vi "Run Bfr Tx - Handle Transmit.vi"(6 "Bytes to Transmit":i32, 7 "Echo Resources in":T1, 8 "error in (no error)":errorcluster, 9 "Runtime Resources":T5={"Connection ID"=refnum, "Transmit Option"=enum."Always", "Destination IP Address"=0, "Destination Port"=0, "Multicast IP Address"=0, "TTL"=0, "Multicast"=FALSE, "Port as Channel"=FALSE, "ExecutionConfig"={"Loop Period"=0, "RT Loop Period"=-2, "Untimed Period"=0, "Target Processor"=0, "Priority"=0, "Thread Management"=enum."Untimed (Default)"}}, 10 "Buffer Resources":T3 {"Data Buffer" format="%016x"}, 11 "Buffer Option Support in":T9) -> (0 "error out":errorcluster, 4 "Tx Packet":string, 5 "Echo Resources out":T1)   [LabVIEW 2019, in "UDP-Custom-Device Engine.lvlib"]
uses:
  UDP-Custom-Device Engine.lvlib
  Types/Engine - Buffered Tx Buffer Option Support.ctl
  Shared/Types/Shared - Transmit Buffer Options.ctl
  Shared/Types/Shared - Transmit Sim Options.ctl
  Types/Engine - Tx Runtime Resources.ctl
  Shared/Types/Shared - Transmit Flag Options.ctl
  Types/Engine - Execution Config.ctl
  Shared/Types/Shared - Thread Management.ctl
  Types/Engine - Buffer Resources.ctl
  Shared/Types/Shared - Pointer Encoding.ctl
  Types/Engine - Tx Echo Resources.ctl
  Shared/Types/Shared - Transmit Echo Options.ctl
  <vilib>/NI VeriStand/VeriStand Data/Pointer Operations/Pointer.In-Place Read (1D U8).vi
  <vilib>/NI VeriStand/VeriStand Data/Pointer Operations/Pointer.Read.vi
  <vilib>/NI VeriStand/VeriStand Data/Pointer Operations/Pointer.Read (I32).vi
  <vilib>/NI VeriStand/VeriStand Data/Pointer Operations/Pointer.Read (U16).vi
  <vilib>/NI VeriStand/VeriStand Data/Pointer Operations/Pointer.In-Place Read (I32).vi
  <vilib>/NI VeriStand/VeriStand Data/Pointer Operations/Pointer.In-Place Read (U16).vi
  <vilib>/NI VeriStand/VeriStand Data/VeriStand Data.lvlib
  Shared/UDP-Custom-Device Shared.lvlib
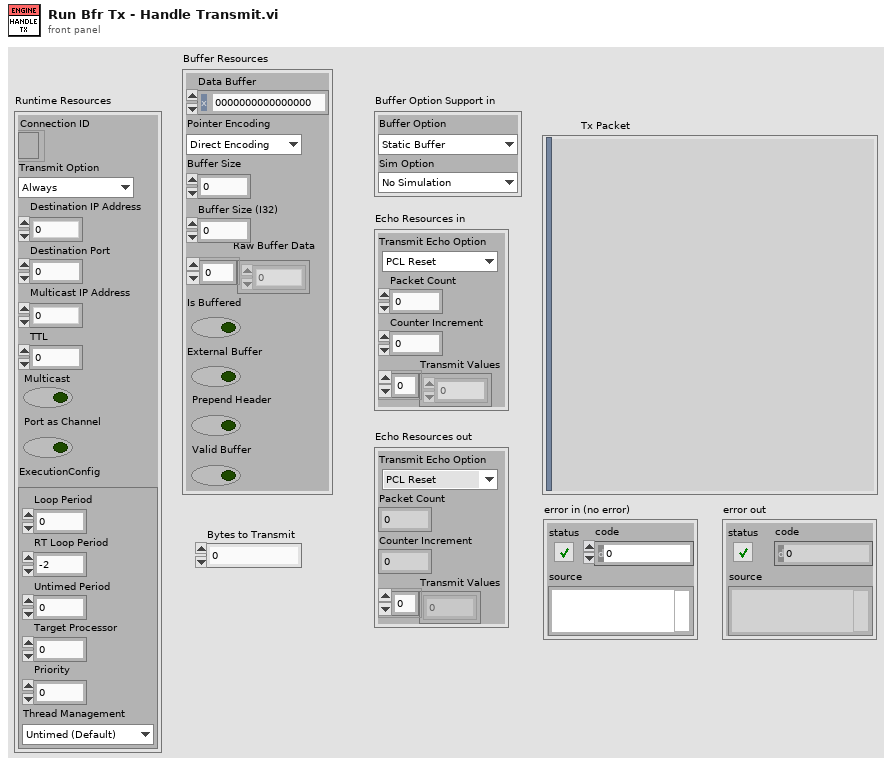
[diagram p1: front panel]
types:
  T1 = typedef "UDP-Custom-Device Engine.lvlib/Engine - Tx Echo Resources.ctl" = cluster{"Transmit Echo Option":T2, "Packet Count":dbl, "Counter Increment":dbl, "Transmit Values":dbl[]}
  T2 = typedef "UDP-Custom-Device Shared.lvlib/Shared - Transmit Echo Options.ctl" = enum16{"PCL Reset", "Counter", "Mirror"}
  T3 = typedef "UDP-Custom-Device Engine.lvlib/Engine - Buffer Resources.ctl" = cluster{"Data Buffer":u64, "Pointer Encoding":T4, "Buffer Size":u64, "Buffer Size (I32)":i32, "Raw Buffer Data":u8[], "Is Buffered":bool, "External Buffer":bool, "Prepend Header":bool, "Valid Buffer":bool}
  T4 = typedef "UDP-Custom-Device Shared.lvlib/Shared - Pointer Encoding.ctl" = enum16{"Direct Encoding", "Conversion Encoding"}
  T5 = typedef "UDP-Custom-Device Engine.lvlib/Engine - Tx Runtime Resources.ctl" = cluster{"Connection ID":refnum<k16>, "Transmit Option":T6, "Destination IP Address":u32, "Destination Port":u16, "Multicast IP Address":u32, "TTL":u16, "Multicast":bool, "Port as Channel":bool, "ExecutionConfig":T7}
  T6 = typedef "UDP-Custom-Device Shared.lvlib/Shared - Transmit Flag Options.ctl" = enum16{"Always", "One-Shot", "Toggle"}
  T7 = typedef "UDP-Custom-Device Engine.lvlib/Engine - Execution Config.ctl" = cluster{"Loop Period":i64, "RT Loop Period":i64, "Untimed Period":u32, "Target Processor":i32, "Priority":i32, "Thread Management":T8}
  T8 = typedef "UDP-Custom-Device Shared.lvlib/Shared - Thread Management.ctl" = enum16{"Untimed (Default)", "Timed (High Priority)"}
  T9 = typedef "UDP-Custom-Device Engine.lvlib/Engine - Buffered Tx Buffer Option Support.ctl" = cluster{"Buffer Option":T10, "Sim Option":T11}
  T10 = typedef "UDP-Custom-Device Shared.lvlib/Shared - Transmit Buffer Options.ctl" = enum16{"Static Buffer", "FIFO Buffer", "FIFO Buffer + Port"}
  T11 = typedef "UDP-Custom-Device Shared.lvlib/Shared - Transmit Sim Options.ctl" = enum16{"No Simulation", "Counter", "Full Buffer", "FIFO Test", "FIFO + Port Test"}
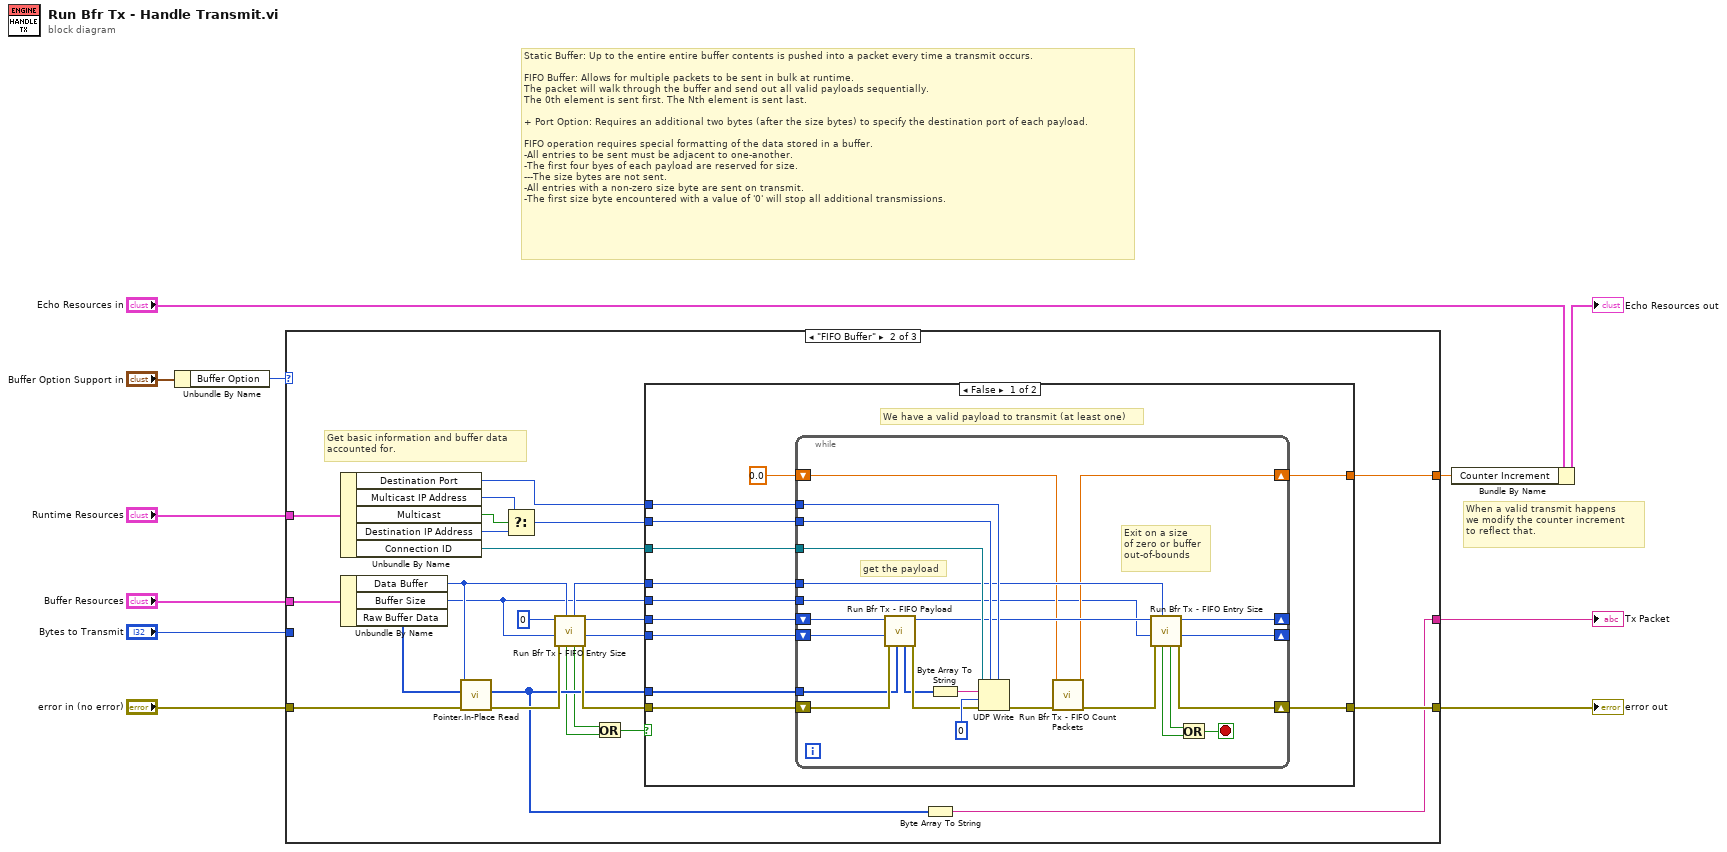
[diagram p0: block diagram]
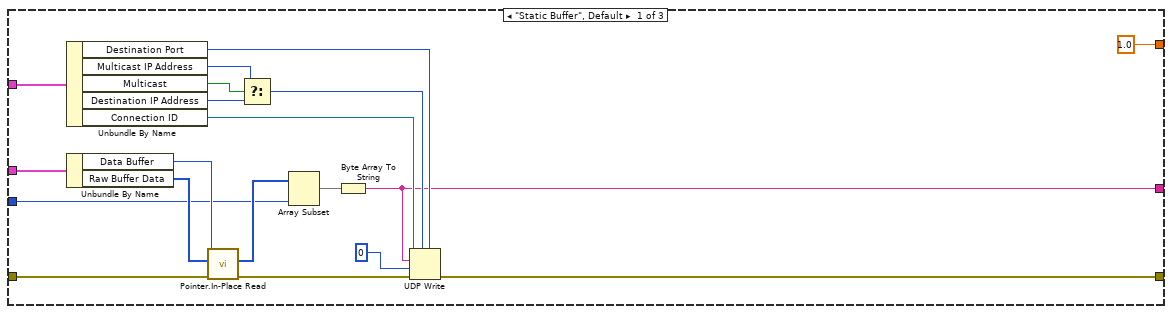
[diagram p2: hidden frame]
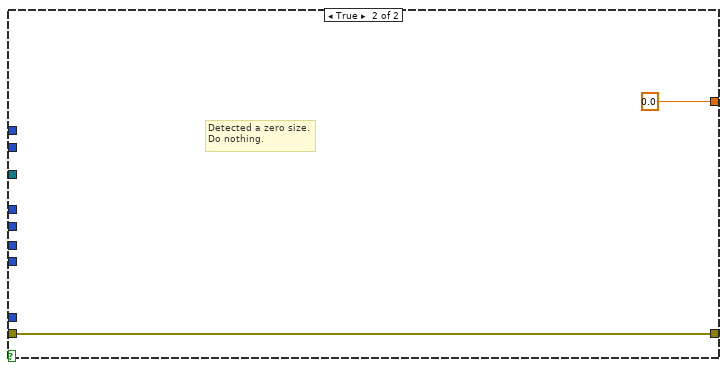
[diagram p3: hidden frame]
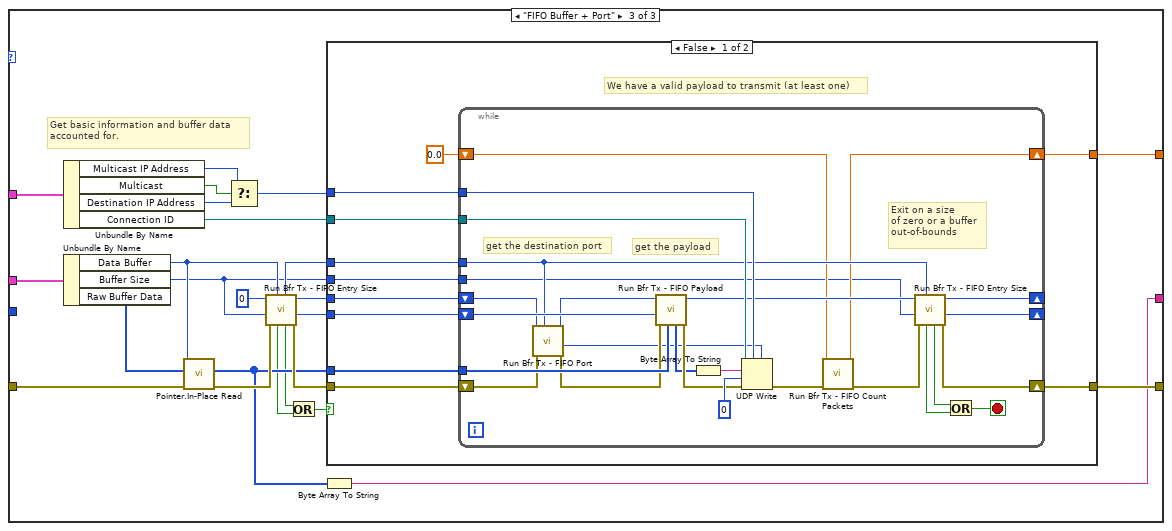
[diagram p4: hidden frame]
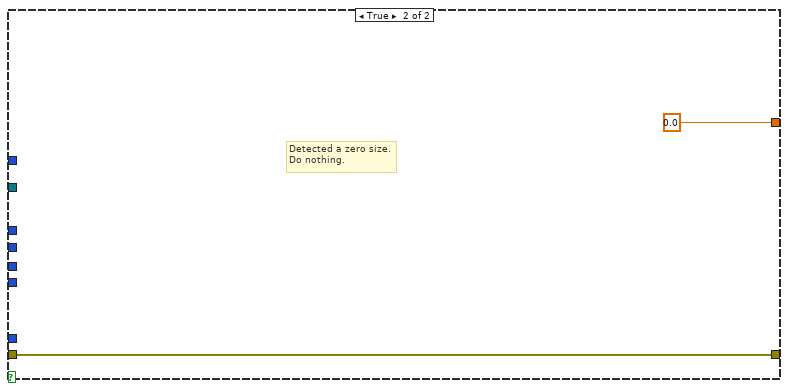
[diagram p5: hidden frame]
diagram:
  # "When a valid transmit happens\nwe modify the counter increment\nto reflect that."
  # "Static Buffer: Up to the entire entire buffer contents is pushed into a packet every time a transmit occurs.\n\nFIFO Buffer: Allows for multiple packets to be sent in bulk at runtime.\nThe packet will walk through the buffer and send out all valid payloads sequentially. \nThe 0th element is sent first. The Nth element is sent last.\n\n+ Port Option: Requires an additional two bytes (after the size bytes) to specify the destination port of each payload.\n\nFIFO operation requires special formatting of the data stored in a buffer.\n-All entries to be sent must be adjacent to one-another.\n-The first four byes of each payload are reserved for size.\n---The size bytes are not sent. \n-All entries with a non-zero size byte are sent on transmit.\n-The first size byte encountered with a value of '0' will stop all additional transmissions."
  n1 = Unbundle By Name("Buffer Option Support in") -> ("Buffer Option"=w4:T10)
  n2 = case shown="\"FIFO Buffer\"" w4 {
    tunnel: "error in (no error)" -> [w18 w47 w110]
    tunnel: "Runtime Resources" -> [w27 w53 w115]
    tunnel: "Buffer Resources" -> [w25 w51 w113]
    tunnel: [w16 w52 w114] -> w8
    tunnel: "Bytes to Transmit" -> [w15 _ _]
    tunnel: [w14 w35 w98] -> w6
    tunnel: [1.0 w37 w100] -> w2
    frame "Static Buffer", Default {
      n3 = Unbundle By Name(w27) -> ("Destination Port"=w22:u16, "Multicast IP Address"=w20:u32, "Multicast"=w13:bool, "Destination IP Address"=w19:u32, "Connection ID"=w26:refnum<k16>)
      n4 = Unbundle By Name(w25) -> ("Data Buffer"=w24:u64, "Raw Buffer Data"=w23:u8[])
      n5 = call-poly <vilib>:"Pointer.In-Place Read.vi"("error in (no error)"=w18, "allocated array in"=w23, "pointer in"=w24) -> ("error out"=w17:errorcluster, "array out"=w30:u8[])  [unwired: 6 in, 1 out]
      n6 = Select(t=w20, s=w13, f=w19) -> (s? t:f=w21:u32)
      n7 = Array Subset(array=w30, length=w15) -> (w29:u8[])  [unwired: 1 in]
      n8 = Byte Array To String(unsigned byte array=w29) -> (string=w14:string)
      n9 = UDP Write(address=w21, port or service name=w22, connection ID=w26, data in=w14, 8:w17, 9:0 ("timeout ms (25000)")) -> (error out=w16:errorcluster)  [unwired: 1 out]
    }
    frame "FIFO Buffer" {
      # "Get basic information and buffer data\naccounted for."
      n10 = Unbundle By Name(w53) -> ("Destination Port"=w49:u16, "Multicast IP Address"=w55:u32, "Multicast"=w38:bool, "Destination IP Address"=w54:u32, "Connection ID"=w50:refnum<k16>)
      n11 = Unbundle By Name(w51) -> ("Data Buffer"=w43:u64, "Buffer Size"=w34:u64, "Raw Buffer Data"=w46:u8[])
      n12 = call-poly <vilib>:"Pointer.In-Place Read.vi"("error in (no error)"=w47, "allocated array in"=w46, "pointer in"=w43) -> ("error out"=w45:errorcluster, "array out"=w36:u8[])  [unwired: 6 in, 1 out]
      n13 = Select(t=w55, s=w38, f=w54) -> (s? t:f=w48:u32)
      n14 = call "Run Bfr Tx - FIFO Entry Size.vi"("Buffer in"=w43, "error in (no error)"=w45, "Buffer Size"=w34, "Offset in"=u64 0) -> ("error out"=w44:errorcluster, "Data Size"=w39:i32, "Offset out"=w40:u64, "Zero Size Detected"=w32:bool, "Buffer out"=w42:u64, "OOB Detected"=w33:bool)  [unwired: 2 in]
      n15 = Or(x=w32, y=w33) -> (x .or. y?=w31:bool)
      n16 = case shown="False" w31 {
        tunnel: [w67 w93] -> w52
        tunnel: w50 -> [w66 _]
        tunnel: w49 -> [w65 _]
        tunnel: w48 -> [w64 _]
        tunnel: w44 -> [w63 w93]
        tunnel: w42 -> [w62 _]
        tunnel: w40 -> [w61 _]
        tunnel: w36 -> [w60 _]
        tunnel: w39 -> [w59 _]
        tunnel: [w57 0.0] -> w37
        tunnel: w34 -> [w56 _]
        frame False {
          # "We have a valid payload to transmit (at least one)"
          n17 = while {
            tunnel: w66 -> [w88]
            tunnel: w65 -> [w90]
            tunnel: w64 -> [w89]
            tunnel: w62 -> [w87]
            shift-right: [w85] -> _
            shift-left: w61 -> [w83]
            tunnel: w60 -> [w78]
            shift-right: [w84] -> _
            shift-left: w59 -> [w81]
            shift-right: [w73] -> w57
            shift-left: 0.0 -> [w74]
            shift-right: [w86] -> w67
            shift-left: w63 -> [w80]
            tunnel: w56 -> [w71]
            stop <- w68 stop-if-true
            # "get the payload"
            # "Exit on a size\nof zero or buffer\nout-of-bounds"
            n18 = call "Run Bfr Tx - FIFO Payload.vi"("Data in"=w78, "error in (no error)"=w80, "Data Size"=w81, "Offset in"=w83) -> ("error out"=w79:errorcluster, "Offset out"=w82:u64, "Data out"=w77:u8[])  [unwired: 5 in]
            n19 = Byte Array To String(unsigned byte array=w77) -> (string=w72:string)
            n20 = UDP Write(address=w89, port or service name=w90, connection ID=w88, data in=w72, 8:w79, 9:0 ("timeout ms (25000)")) -> (error out=w76:errorcluster)  [unwired: 1 out]
            n21 = call "Run Bfr Tx - FIFO Count Packets.vi"("error in (no error)"=w76, "Packet Count (t-1)"=w74) -> ("error out"=w75:errorcluster, "Packet Count (t)"=w73:dbl)  [unwired: 8 in]
            n22 = call "Run Bfr Tx - FIFO Entry Size.vi"("Buffer in"=w87, "error in (no error)"=w75, "Buffer Size"=w71, "Offset in"=w82) -> ("error out"=w86:errorcluster, "Data Size"=w84:i32, "Offset out"=w85:u64, "Zero Size Detected"=w70:bool, "OOB Detected"=w69:bool)  [unwired: 2 in, 1 out]
            n23 = Or(x=w70, y=w69) -> (x .or. y?=w68:bool)
          }
        }
        frame True {
          # "Detected a zero size.\nDo nothing."
        }
      }
      n24 = Byte Array To String(unsigned byte array=w36) -> (string=w35:string)
    }
    frame "FIFO Buffer + Port" {
      # "Get basic information and buffer data\naccounted for."
      n25 = Unbundle By Name(w115) -> ("Multicast IP Address"=w117:u32, "Multicast"=w101:bool, "Destination IP Address"=w116:u32, "Connection ID"=w112:refnum<k16>)
      n26 = Unbundle By Name(w113) -> ("Data Buffer"=w106:u64, "Buffer Size"=w97:u64, "Raw Buffer Data"=w109:u8[])
      n27 = call-poly <vilib>:"Pointer.In-Place Read.vi"("error in (no error)"=w110, "allocated array in"=w109, "pointer in"=w106) -> ("error out"=w108:errorcluster, "array out"=w99:u8[])  [unwired: 6 in, 1 out]
      n28 = Select(t=w117, s=w101, f=w116) -> (s? t:f=w111:u32)
      n29 = call "Run Bfr Tx - FIFO Entry Size.vi"("Buffer in"=w106, "error in (no error)"=w108, "Buffer Size"=w97, "Offset in"=u64 0) -> ("error out"=w107:errorcluster, "Data Size"=w102:i32, "Offset out"=w103:u64, "Zero Size Detected"=w95:bool, "Buffer out"=w105:u64, "OOB Detected"=w96:bool)  [unwired: 2 in]
      n30 = Or(x=w95, y=w96) -> (x .or. y?=w94:bool)
      n31 = Byte Array To String(unsigned byte array=w99) -> (string=w98:string)
      n32 = case shown="False" w94 {
        tunnel: [w128 w156] -> w114
        tunnel: w112 -> [w127 _]
        tunnel: w111 -> [w126 _]
        tunnel: w107 -> [w125 w156]
        tunnel: w105 -> [w124 _]
        tunnel: w103 -> [w123 _]
        tunnel: w99 -> [w122 _]
        tunnel: w102 -> [w121 _]
        tunnel: [w119 0.0] -> w100
        tunnel: w97 -> [w118 _]
        frame False {
          # "We have a valid payload to transmit (at least one)"
          n33 = while {
            tunnel: w127 -> [w152]
            tunnel: w126 -> [w153]
            tunnel: w124 -> [w140]
            shift-right: [w150] -> _
            shift-left: w123 -> [w142]
            tunnel: w122 -> [w145]
            shift-right: [w149] -> _
            shift-left: w121 -> [w147]
            shift-right: [w135] -> w119
            shift-left: 0.0 -> [w136]
            shift-right: [w151] -> w128
            shift-left: w125 -> [w139]
            tunnel: w118 -> [w132]
            stop <- w129 stop-if-true
            # "get the destination port"
            # "get the payload"
            # "Exit on a size\nof zero or a buffer\nout-of-bounds"
            n34 = call "Run Bfr Tx - FIFO Port.vi"("Buffer in"=w140, "error in (no error)"=w139, "Offset in"=w142) -> ("error out"=w138:errorcluster, "Dest Port"=w137:u16, "Offset out"=w141:u64)  [unwired: 5 in, 1 out]
            n35 = call "Run Bfr Tx - FIFO Payload.vi"("Data in"=w145, "error in (no error)"=w138, "Data Size"=w147, "Offset in"=w141) -> ("error out"=w146:errorcluster, "Offset out"=w148:u64, "Data out"=w143:u8[])  [unwired: 5 in]
            n36 = Byte Array To String(unsigned byte array=w143) -> (string=w144:string)
            n37 = UDP Write(address=w153, port or service name=w137, connection ID=w152, data in=w144, 8:w146, 9:0 ("timeout ms (25000)")) -> (error out=w134:errorcluster)  [unwired: 1 out]
            n38 = call "Run Bfr Tx - FIFO Count Packets.vi"("error in (no error)"=w134, "Packet Count (t-1)"=w136) -> ("error out"=w133:errorcluster, "Packet Count (t)"=w135:dbl)  [unwired: 8 in]
            n39 = call "Run Bfr Tx - FIFO Entry Size.vi"("Buffer in"=w140, "error in (no error)"=w133, "Buffer Size"=w132, "Offset in"=w148) -> ("error out"=w151:errorcluster, "Data Size"=w149:i32, "Offset out"=w150:u64, "Zero Size Detected"=w131:bool, "OOB Detected"=w130:bool)  [unwired: 2 in, 1 out]
            n40 = Or(x=w131, y=w130) -> (x .or. y?=w129:bool)
          }
        }
        frame True {
          # "Detected a zero size.\nDo nothing."
        }
      }
    }
  }
  "error out" <- w8
  "Tx Packet" <- w6
  n41 = Bundle By Name(cluster="Echo Resources in", "Counter Increment"=w2) -> (→"Echo Resources out":T1)
